vi "RoundToHalfPositions.vi"(11 "input cluster":T1) -> (3 "output cluster":T1)   [LabVIEW 2014, in "Manipulator.lvclass"]
uses:
  Manipulator.lvclass
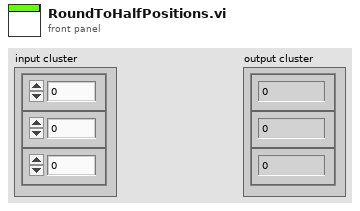
[diagram p1: front panel]
types:
  T1 = cluster{"Numeric Control":dbl, "Numeric Control":dbl, "Numeric Control":dbl}
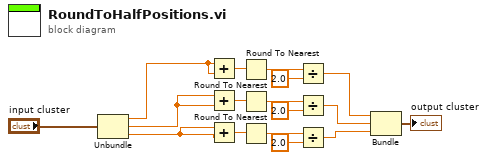
[diagram p0: block diagram]
diagram:
  n1 = Unbundle("input cluster") -> ("Numeric Control"=w5:dbl, "Numeric Control"=w4:dbl, "Numeric Control"=w3:dbl)
  n2 = Add(x=w5, y=w5) -> (x+y=w15:dbl)
  n3 = Add(x=w4, y=w4) -> (x+y=w13:dbl)
  n4 = Add(x=w3, y=w3) -> (x+y=w7:dbl)
  n5 = Round To Nearest(number=w15) -> (nearest integer value=w16:dbl)
  n6 = Round To Nearest(number=w13) -> (nearest integer value=w12:dbl)
  n7 = Round To Nearest(number=w7) -> (nearest integer value=w8:dbl)
  n8 = Divide(x=w16, y=2.0) -> (x/y=w14:dbl)
  n9 = Divide(x=w12, y=2.0) -> (x/y=w10:dbl)
  n10 = Divide(x=w8, y=2.0) -> (x/y=w6:dbl)
  n11 = Bundle(w14, w10, w6) -> (→"output cluster":cluster{dbl, dbl, dbl})  [unwired: 1 in]
